vi "SPI IRQ.vi"(9 "SPI.A.IRQ.NO":u8=15, 10 "SPI.STAT":u8, 11 "FIFO In":refnum<k21>="DIO A IRQ") -> ()   [LabVIEW 2017]
uses:
  <vilib>/rvi/eio/common/nirviEmuReportErrorAndStop.vi
  <vilib>/rvi/interface/RandomDataEmulation/niFpgaRandomDataHandleErrors.vi
  <vilib>/rvi/Emulation/niFpgaProcessEmulError.vi
  <vilib>/rvi/FIFO/Fifo_Resource/nirvififoEmulationSetSize.vi
  <vilib>/rvi/DataTransferAndStorage/Container/Common/niFpgaContainerGetUniqueNameForEmu.vi
  <vilib>/rvi/FIFO/Fifo_Resource/nirviFifoEmulationQueueMgr.vi
  <instcachedir>/0/nirviFifoEmulationQueueMgr_E5CAEC123FF24DC58D834DCA3CDAA9B5.lvgen/nirviFifoEmulationQueueMgr_E5CAEC123FF24DC58D834DCA3CDAA9B5_001.vi
  <vilib>/rvi/Emulation/niFpgaEmulationIsFPGAContextNoSignature.vi
  <vilib>/rvi/errors/nirviReportUnexpectedCaseInternalError.vi
  <vilib>/rvi/errors/nirviReportUnexpectedCaseInternalError (U32).vi
  <vilib>/rvi/occurrence/nirviWaitOnOccurrenceBase.vi
  <vilib>/rvi/FIFO/Fifo_Resource/nirvififoEmulationReleaseLock.vi
  <vilib>/rvi/FIFO/Fifo_Resource/nirvififoEmulationObtainLock.vi
  <vilib>/rvi/FIFO/Fifo_Resource/nirvififoEmulationCreateLock.vi
  <vilib>/Utility/error.llb/Clear Errors.vi
  <vilib>/rvi/errors/niFpgaSetErrorForExecOnDevCompSimple.vi
  <vilib>/rvi/Emulation/niFpgaSctlEmulationGetInTimedLoop.vi
  <vilib>/rvi/FIFO/Fifo_Resource/nirvififoEmulationDetermineInputValidOut.vi
  <vilib>/rvi/DataTransferAndStorage/Container/Common/niFpgaContainerExecOnDevCompGetState.vi
  <vilib>/rvi/DataTransferAndStorage/Container/XNode/niFpgaContainer.xnode
  <vilib>/rvi/FIFO/Fifo_Resource/niFpgaFifoEmulationRefIn.vi
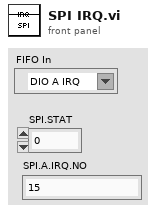
[diagram p1: front panel]
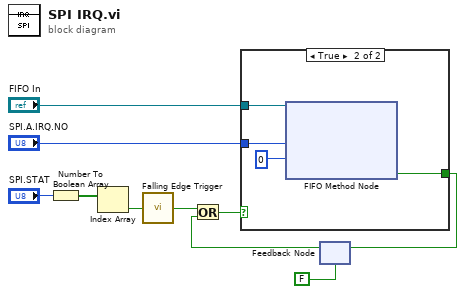
[diagram p0: block diagram]
diagram:
  n1 = Number To Boolean Array(number="SPI.STAT") -> (Boolean array=w10:bool[])
  n2 = Index Array(array=w10) -> (element=w9:bool)  [unwired: 1 in]
  n3 = call "Falling Edge Trigger.vi"("Signal"=w9) -> ("Trigger?"=w5:bool)
  n4 = feedback #1(FALSE ("Timed Out?")) -> (w1:bool)
  n5 = Or(x=w5, y=w1) -> (x .or. y?=w4:bool)
  n6 = case shown="True" w4 {
    selector: w4 -> [w11 _]
    tunnel: "FIFO In" -> [_ w15]
    tunnel: "SPI.A.IRQ.NO" -> [_ w14]
    tunnel: [w11 w12] -> w2
    frame False {
    }
    frame True {
      n7 = xnode ("FIFO Method Node")("Element"=w14, "Timeout"=0, "FIFO In"=w15) -> ("Timed Out?"=w12:bool)  [unwired: 1 out]
    }
  }
  n8 = feedback-in #1(w2) -> ()
